vi "Parse Tokens.vi"(8 "Error In":errorcluster, 10 "Tokens":refnum<class "Token.lvclass">[](array[class]), 11 "Stack In":refnum<queue>) -> (0 "Error Out":errorcluster, 3 "Stack Out":refnum<queue>)   [LabVIEW 2018, in "Toolkit.lvlib" / "Parser.lvclass"]
uses:
  Parser.lvclass
  Nodes/NonTerminal/NonTerminal.lvclass
  Tokens/Token/Token.lvclass
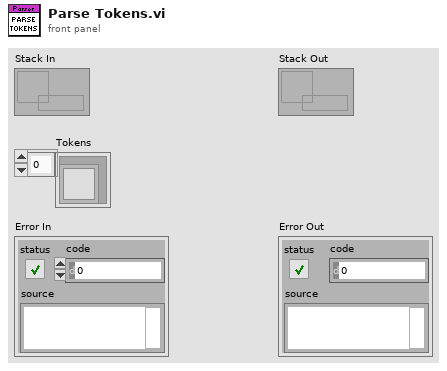
[diagram p1: front panel]
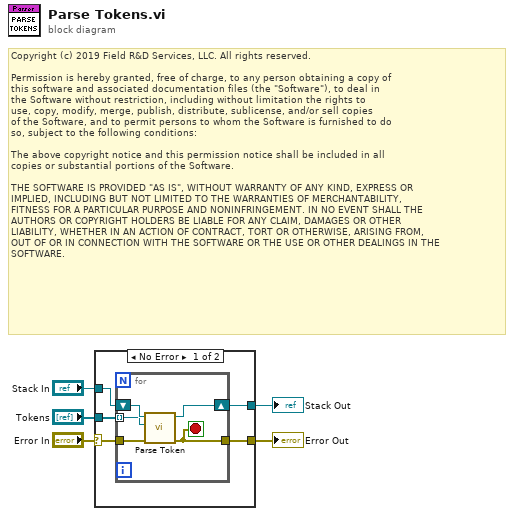
[diagram p0: block diagram]
diagram:
  # "Copyright (c) 2019 Field R&D Services, LLC. All rights reserved.\n\nPermission is hereby granted, free of charge, to any person obtaining a copy of\nthis software and associated documentation files (the \"Software\"), to deal in\nthe Software without restriction, including without limitation the rights to\nuse, copy, modify, merge, publish, distribute, sublicense, and/or sell copies\nof the Software, and to permit persons to whom the Software is furnished to do\nso, subject to the following conditions:\n\nThe above copyright notice and this permission notice shall be included in all\ncopies or substantial portions of the Software.\n\nTHE SOFTWARE IS PROVIDED \"AS IS\", WITHOUT WARRANTY OF ANY KIND, EXPRESS OR\nIMPLIED, INCLUDING BUT NOT LIMITED TO THE WARRANTIES OF MERCHANTABILITY,\nFITNESS FOR A PARTICULAR PURPOSE AND NONINFRINGEMENT. IN NO EVENT SHALL THE\nAUTHORS OR COPYRIGHT HOLDERS BE LIABLE FOR ANY CLAIM, DAMAGES OR OTHER\nLIABILITY, WHETHER IN AN ACTION OF CONTRACT, TORT OR OTHERWISE, ARISING FROM,\nOUT OF OR IN CONNECTION WITH THE SOFTWARE OR THE USE OR OTHER DEALINGS IN THE\nSOFTWARE."
  n1 = case shown="No Error" "Error In" {
    selector: "Error In" -> [w6 w16]
    tunnel: [w10 w17] -> w5
    tunnel: "Stack In" -> [w9 w17]
    tunnel: "Tokens" -> [w8 _]
    tunnel: [w7 w16] -> w2
    frame No Error {
      n2 = for {
        tunnel: w8 -> [w11] mode=indexing
        tunnel: w6 -> [w15]
        tunnel: [w14] -> w7
        shift-right: [w13] -> w10
        shift-left: w9 -> [w12]
        stop <- w14 stop-if-true
        n3 = call "Parse Token.vi"("Error In"=w15, "Token"=w11, "Stack In"=w12) -> ("Error Out"=w14:errorcluster, "Stack Out"=w13:refnum<queue>)  [unwired: 7 in]
      }
    }
    frame Error {
    }
  }
  "Stack Out" <- w5
  "Error Out" <- w2
